vi "Create Function String (Current).vi"(8 "error in (no error)":errorcluster, 9 "Element (1: 1)":i32(ring)=1 items=["Null", "1", "2", "3", "Sigma A"], 10 "Function (0: I)":i32(ring) items=["I", "IPPeak", "IMPeak"], 11 "VISA resource name":refnum<visa-resource-name>) -> (0 "error out":errorcluster, 2 "Function String":string, 3 "VISA resource name out":refnum<visa-resource-name>)   [LabVIEW 2016, in "Yokogawa WT300 Series.lvlib"]
doc: "Create a current function string"
uses:
  Yokogawa WT300 Series.lvlib
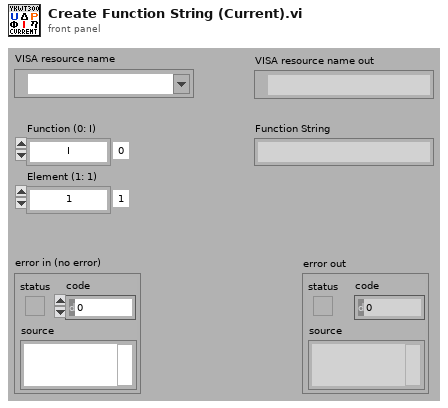
[diagram p1: front panel]
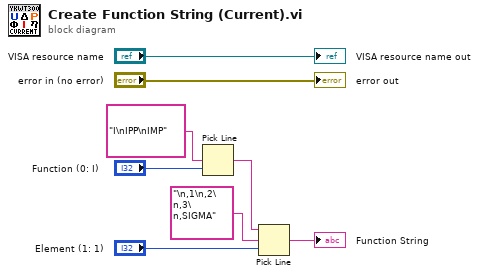
[diagram p0: block diagram]
diagram:
  n1 = Pick Line ("ライン選択")(multi-line string="I\nIPP\nIMP" ("複数行文字列"), line index="Function (0: I)") -> (output string=w4:string)  [unwired: 1 in]
  n2 = Pick Line ("ライン選択")(string ("")=w4, multi-line string="\n,1\n,2\n,3\n,SIGMA" ("複数行文字列"), line index="Element (1: 1)") -> (output string=→"Function String":string)
  "VISA resource name out" <- "VISA resource name"
  "error out" <- "error in (no error)"
